vi "generate table.vi"(4 "only redraw current":bool, 6 "select last?":bool, 8 "error in":errorcluster, 9 "listbox":refnum<vi>, 10 "engine configuration in":refnum<class "engine configuration.lvclass">, 11 "tag bus configurable plugin module configuration in":refnum<class "tag bus processing plugin module configuration.lvclass">) -> (0 "error out":errorcluster)   [LabVIEW 2013, in "tag bus processing plugin editor node.lvclass"]
uses:
  tag bus processing plugin editor node.lvclass
  module/configuration/tag bus processing plugin module configuration.lvclass
  <vilib>/NI/Module Execution Interface/Engine Configuration/engine configuration.lvclass
  <vilib>/NI/Tag Bus Module Framework/root configuration/TBM configuration.lvclass/TBM configuration.ctl
  module/configuration/tag bus processing plugin module configuration.lvclass/tag bus processing plugin module configuration.ctl
  <vilib>/NI/Tag Bus Module Framework/root configuration/Read instance name.vi
  module/configuration/Read functions.vi
  <vilib>/NI/Tag Bus Module Framework/root configuration/create GUID.vi
  <vilib>/NI/Tag Bus Module Framework/channel/TBM channel.lvclass
panel:
  in  "reverse list":bool
  in  "sort?":bool
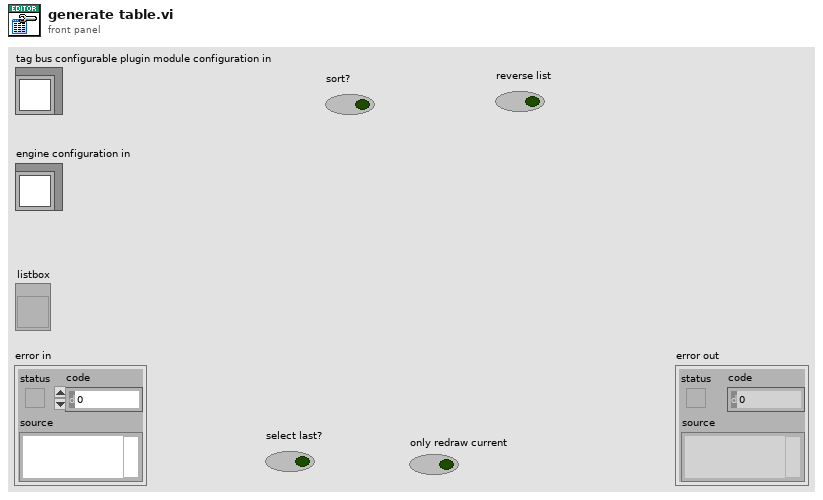
[diagram p1: front panel]
types:
  T1 = typedef "tag bus processing plugin module configuration.lvclass/processing channels.ctl" = cluster{"parameter":refnum<class "TBM channel.lvclass">, "result":refnum<class "TBM channel.lvclass">}
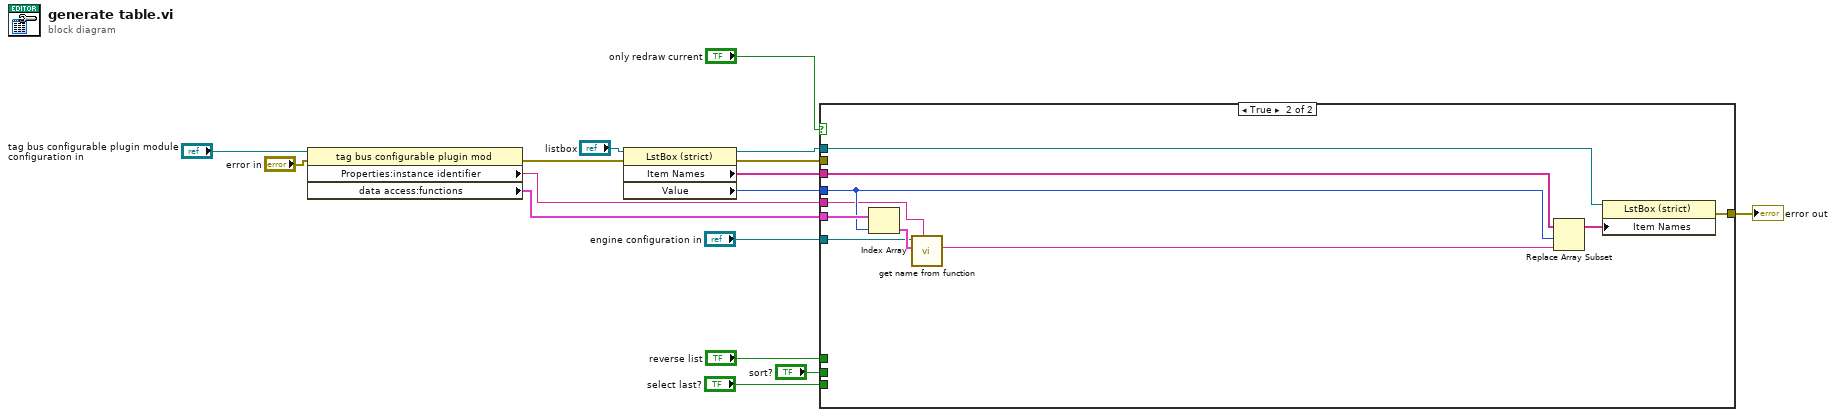
[diagram p0: block diagram]
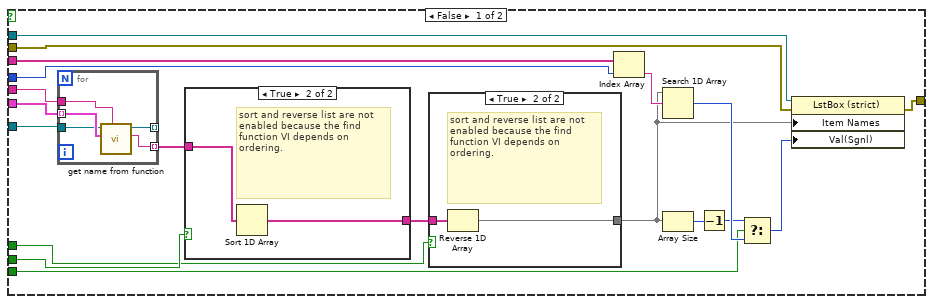
[diagram p2: hidden frame]
diagram:
  n1 = property class="tag bus configurable plugin mod"(reference="tag bus configurable plugin module configuration in", error in="error in") -> (error out=w3:errorcluster, "Properties:instance identifier"=w10:string, "data access:functions"=w13:T1[])  [unwired: 1 out]
  n2 = property class="LstBox (strict)"(reference="listbox", error in=w3) -> (reference out=w7:refnum<vi>, error out=w8:errorcluster, "Item Names"=w6:string[], "Value"=w5:i32)
  n3 = case shown="True" "only redraw current" {
    tunnel: [w35 w55] -> w14
    tunnel: w13 -> [w34 w54]
    tunnel: "sort?" -> [w33 _]
    tunnel: "reverse list" -> [w32 _]
    tunnel: w10 -> [w29 w48]
    tunnel: "engine configuration in" -> [w28 w49]
    tunnel: w8 -> [w27 _]
    tunnel: w7 -> [w26 w56]
    tunnel: w6 -> [w25 w53]
    tunnel: w5 -> [w24 w51]
    tunnel: "select last?" -> [w20 _]
    frame False {
      n4 = for {
        tunnel: w34 -> [w46] mode=indexing
        tunnel: [w44] -> w31 mode=indexing
        tunnel: w29 -> [w45]
        tunnel: w28 -> [w42]
        tunnel: [w43] -> _ mode=indexing
        n5 = call "get name from function.vi"("owner"=w45, "processing function"=w46, "engine configuration in"=w42) -> ("name"=w44:string, "engine configuration out"=w43:refnum<class "engine configuration.lvclass">)  [unwired: 7 in]
      }
      n6 = case shown="True" w33 {
        tunnel: w31 -> [w39 w41]
        tunnel: [w39 w40] -> w30
        frame False {
        }
        frame True {
          # "sort and reverse list are not enabled because the find function VI depends on ordering."
          n7 = Sort 1D Array(array=w41) -> (sorted array=w40:string[])
        }
      }
      n8 = case shown="True" w32 {
        tunnel: [w36 w37] -> w18
        tunnel: w30 -> [w36 w38]
        frame False {
        }
        frame True {
          # "sort and reverse list are not enabled because the find function VI depends on ordering."
          n9 = Reverse 1D Array(array=w38) -> (reversed array=w37:string[])
        }
      }
      n10 = Index Array(array=w25, index=w24) -> (element=w23:string)
      n11 = Search 1D Array(1D array=w18, element=w23) -> (index of element=w22:i32)  [unwired: 1 in]
      n12 = Array Size(array=w18) -> (size(s)=w19:i32)
      n13 = Decrement(x=w19) -> (x-1=w17:i32)
      n14 = Select(t=w17, s=w20, f=w22) -> (s? t:f=w21:i32)
      n15 = property class="LstBox (strict)"(reference=w26, error in=w27, "Item Names"=w18, "Val(Sgnl)"=w21) -> (error out=w35:errorcluster)  [unwired: 1 out]
    }
    frame True {
      n16 = Index Array(array=w54, index=w51) -> (element=w50:T1)
      n17 = call "get name from function.vi"("owner"=w48, "processing function"=w50, "engine configuration in"=w49) -> ("name"=w47:string)  [unwired: 7 in, 1 out]
      n18 = Replace Array Subset(array=w53, new element=w47, index=w51) -> (w52:string[])
      n19 = property class="LstBox (strict)"(reference=w56, "Item Names"=w52) -> (error out=w55:errorcluster)  [unwired: 1 in, 1 out]
    }
  }
  "error out" <- w14
